vi "Find local ipv4Addr.vi"(11 "MachineToFind":string) -> (2 "name":string, 3 "IP Addresses":string[](array[string]))   [LabVIEW 2019]
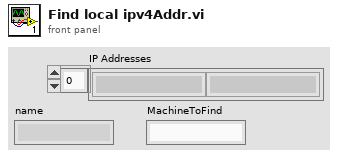
[diagram p1: front panel]
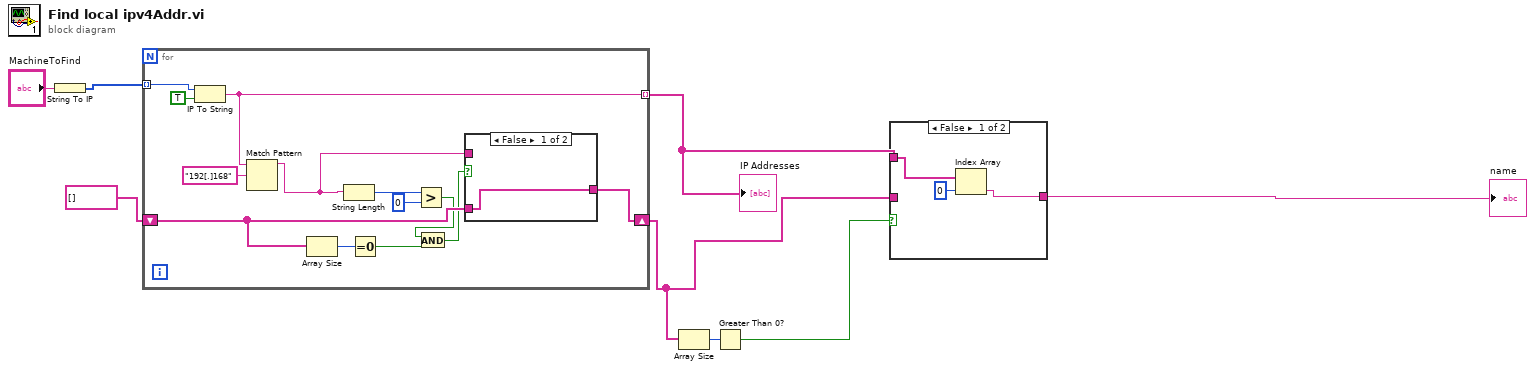
[diagram p0: block diagram]
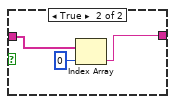
[diagram p2: hidden frame]
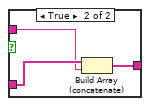
[diagram p3: hidden frame]
diagram:
  n1 = String To IP(1:"MachineToFind") -> (0:w2:u32[])
  n2 = for {
    tunnel: w2 -> [w20] mode=indexing
    tunnel: [w19] -> w7 mode=indexing
    shift-right: [w14] -> w6
    shift-left: string[] [] -> [w13]
    n3 = IP To String(1:TRUE ("dot notation? (F)"), 2:w20) -> (0:w19:string)
    n4 = Match Pattern(string=w19, regular expression="192[.]168") -> (before substring=w15:string)  [unwired: 1 in, 3 out]
    n5 = Array Size(array=w13) -> (size(s)=w12:i32)
    n6 = String Length(string=w15) -> (length=w17:i32)
    n7 = Equal To 0?(x=w12) -> (x = 0?=w11:bool)
    n8 = Greater?(x=w17, y=0) -> (0:w10:bool)
    n9 = And(x=w10, y=w11) -> (x .and. y?=w9:bool)
    n10 = case shown="False" w9 {
      tunnel: w13 -> [w22 w25]
      tunnel: w15 -> [_ w24]
      tunnel: [w22 w23] -> w14
      frame False {
      }
      frame True {
        n11 = Build Array (concatenate)(w25, w24) -> (w23:string[])
      }
    }
  }
  "IP Addresses" <- w7
  n12 = Array Size(array=w6) -> (size(s)=w4:i32)
  n13 = Greater Than 0?(x=w4) -> (x > 0?=w5:bool)
  n14 = case shown="False" w5 {
    tunnel: w6 -> [_ w31]
    tunnel: w7 -> [w28 _]
    tunnel: [w26 w29] -> w8
    frame False {
      n15 = Index Array(array=w28, index=0) -> (element=w26:string)
    }
    frame True {
      n16 = Index Array(array=w31, index=0) -> (element=w29:string)
    }
  }
  "name" <- w8
